vi "Get Multiline Str.vi"(8 "error in":errorcluster, 11 "Serial Session in":refnum<class "Serial Session.lvclass">) -> (0 "error out":errorcluster, 2 "Multiline Str":string, 3 "Serial Session out":refnum<class "Serial Session.lvclass">)   [LabVIEW 2019, in "Serial Session.lvclass"]
doc: "This VI calls the <b>Read</b> method to retrieve multiple lines of data from teh serial device. This VI is intended to relieve resource conflicts (i.e. when on portion of the code sends a request and expects a multiline response but when another attempts to read off of the same port when the initial Read call is returned)."
uses:
  Serial Session.lvclass
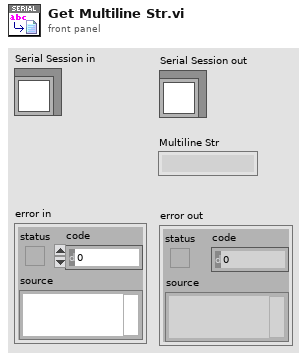
[diagram p1: front panel]
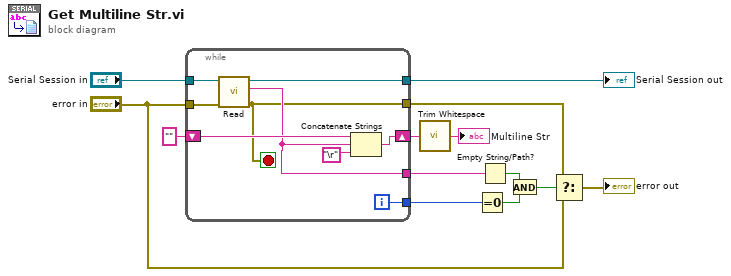
[diagram p0: block diagram]
diagram:
  n1 = while {
    tunnel: "Serial Session in" -> [w22]
    shift-right: [w20] -> w4
    shift-left: "" -> [w19]
    tunnel: [w18] -> w12
    tunnel: [w17] -> w10
    tunnel: [w16] -> w7
    tunnel: "error in" -> [w15]
    tunnel: [w14] -> w1
    i -> [w17]
    stop <- w16 stop-if-true
    n2 = call-dynamic "Read.vi"("error in"=w15, "Serial Session in"=w22) -> ("error out"=w16:errorcluster, "Data Out"=w18:string, "Serial Session out"=w14:refnum<class "Serial Session.lvclass">)  [unwired: 7 in]
    n3 = Concatenate Strings(w19, w18, "\r") -> (w20:string)
  }
  "Serial Session out" <- w1
  n4 = call <vilib>:"Trim Whitespace.vi"("string"=w4) -> ("trimmed string"=→"Multiline Str":string)  [unwired: 1 in]
  n5 = Equal To 0?(x=w10) -> (x = 0?=w9:bool)
  n6 = Empty String/Path?(string/path=w12) -> (empty?=w11:bool)
  n7 = And(x=w11, y=w9) -> (x .and. y?=w8:bool)
  n8 = Select(t=w7, s=w8, f="error in") -> (s? t:f=→"error out":errorcluster)
